vi "Clusters.vi"() -> ()   [LabVIEW 2018]
panel:
  out "Numeric":dbl
  out "Boolean":bool
  out "String":string
  in  "Cluster":cluster{}
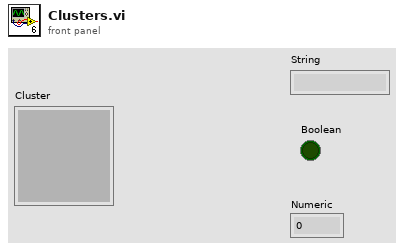
[diagram p1: front panel]
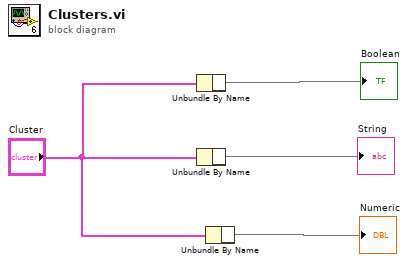
[diagram p0: block diagram]
diagram:
  n1 = Unbundle By Name("Cluster") -> (→"Boolean")
  n2 = Unbundle By Name("Cluster") -> (→"String")
  n3 = Unbundle By Name("Cluster") -> (→"Numeric")
